vi "getState.vi"(8 "error in (no error)":errorcluster, 11 "SetDurationReading in":refnum<class "SetDurationReading.lvclass">) -> (0 "error out":errorcluster, 2 "State":T1=enum."Configuring", 3 "SetDurationReading out":refnum<class "SetDurationReading.lvclass">)   [LabVIEW 2016, in "SetDurationReading.lvclass"]
uses:
  SetDurationReading.lvclass
  internalState.ctl
  Electrometer.lvclass
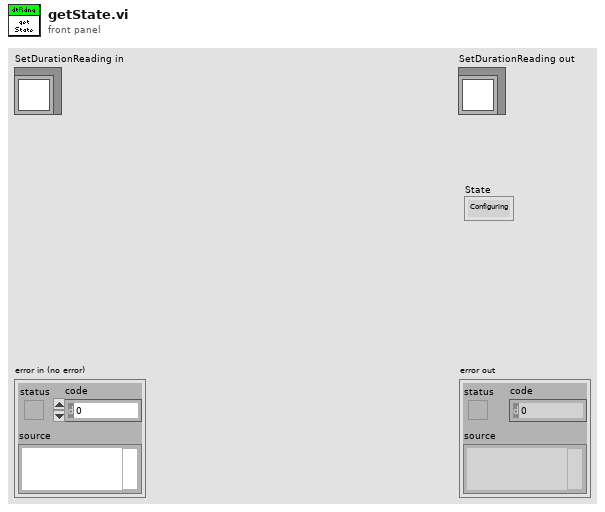
[diagram p1: front panel]
types:
  T1 = typedef "Electrometer.lvclass/internalState.ctl" = enum16{"Ready", "Configuring", "ManualReading", "UntilIntensityReading", "SetDurationReading"}
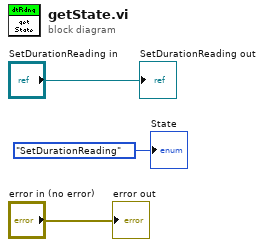
[diagram p0: block diagram]
diagram:
  "error out" <- "error in (no error)"
  "SetDurationReading out" <- "SetDurationReading in"
  "State" <- internalState."SetDurationReading" ("States")
